vi "Start.vi"(0 "Address":string="localhost", 5 "Port":dbl=27015.0, 11 "error in (no error)":errorcluster) -> (4 "TecellaClient":refnum<class "TecellaClient.lvclass">, 6 "isAlive":bool, 8 "Is Simulated?":bool, 10 "Running?":bool, 15 "error out":errorcluster)   [LabVIEW 2009, in "TecellaClient.lvclass"]
uses:
  TecellaClient.lvclass
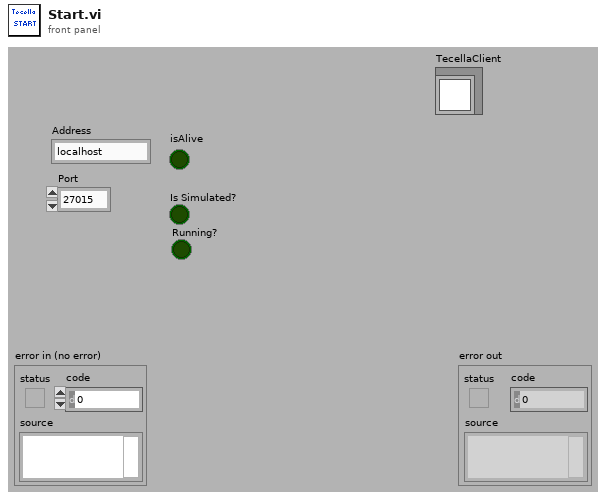
[diagram p1: front panel]
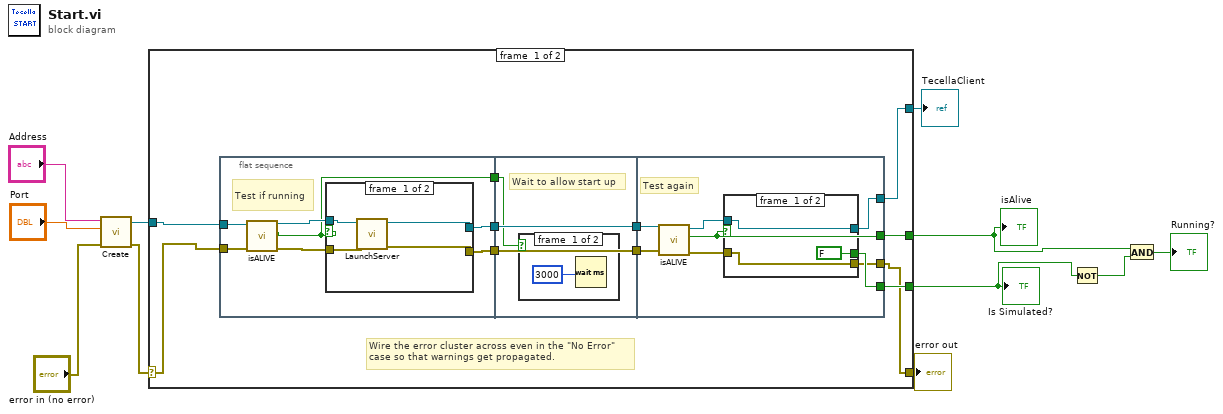
[diagram p0: block diagram]
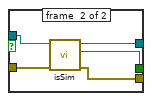
[diagram p4: hidden frame]
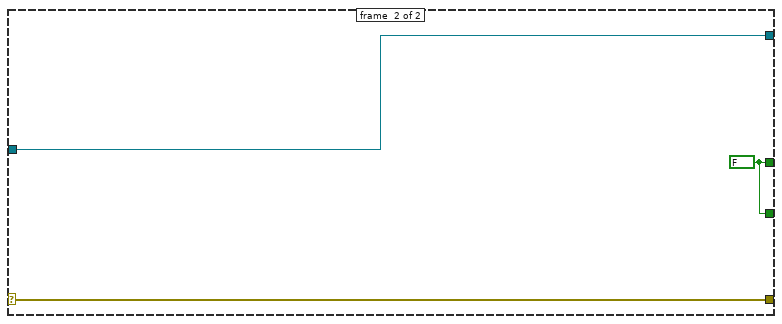
[diagram p5: hidden frame]
diagram:
  n1 = call "Create.vi"("error in (no error)"="error in (no error)", "Port"="Port", "Address"="Address") -> ("error out"=w8:errorcluster, "TecellaClient out"=w9:refnum<class "TecellaClient.lvclass">)  [unwired: 7 in]
  n2 = case shown="No Error" w8 {
    selector: w8 -> [w16 w57]
    tunnel: [w14 w57] -> w11
    tunnel: [w13 w58] -> w10
    tunnel: [w18 w56] -> w5
    tunnel: w9 -> [w17 w58]
    tunnel: [w15 w56] -> w4
    frame #0 {
      # "Wire the error cluster across even in the \"No Error\"\ncase so that warnings get propagated."
      n3 = flat-sequence {
        tunnel: [w29] -> w22
        tunnel: [w28] -> w21
        tunnel: w17 -> [w25]
        tunnel: w16 -> [w24]
        tunnel: [w23] -> w12
        tunnel: w22 -> [w38]
        tunnel: [w38] -> w20
        tunnel: w21 -> [w37]
        tunnel: [w37] -> w19
        tunnel: w12 -> [w36]
        tunnel: [w45] -> w18
        tunnel: w20 -> [w47]
        tunnel: w19 -> [w46]
        tunnel: [w44] -> w15
        tunnel: [w42] -> w14
        tunnel: [w41] -> w13
        frame #0 {
          # "Test if running"
          n4 = call-dynamic "isALIVE.vi"("error in (no error)"=w24, "TecellaClient in"=w25) -> ("error out"=w26:errorcluster, "Boolean"=w23:bool, "TecellaClient out"=w27:refnum<class "TecellaClient.lvclass">)  [unwired: 7 in]
          n5 = case shown="False" w23 {
            tunnel: [w32 w35] -> w29
            tunnel: [w33 w34] -> w28
            tunnel: w27 -> [w31 w35]
            tunnel: w26 -> [w30 w34]
            frame #0 {
              n6 = call-dynamic "LaunchServer.vi"("error in (no error)"=w30, "TecellaClient in"=w31) -> ("error out"=w33:errorcluster, "TecellaClient out"=w32:refnum<class "TecellaClient.lvclass">)  [unwired: 8 in]
            }
            frame #1 {
            }
          }
        }
        frame #1 {
          # "Wait to allow start up"
          n7 = case shown="False" w36 {
            frame #0 {
              n8 = Wait (ms)(milliseconds to wait=u32 3000) -> ()  [unwired: 1 out]
            }
            frame #1 {
            }
          }
        }
        frame #2 {
          # "Test again"
          n9 = call-dynamic "isALIVE.vi"("error in (no error)"=w46, "TecellaClient in"=w47) -> ("error out"=w43:errorcluster, "Boolean"=w45:bool, "TecellaClient out"=w40:refnum<class "TecellaClient.lvclass">)  [unwired: 7 in]
          n10 = case shown="False" w45 {
            tunnel: [FALSE ("Is Simulated?") w55] -> w44
            tunnel: w43 -> [w49 w54]
            tunnel: [w49 w53] -> w42
            tunnel: [w50 w52] -> w41
            tunnel: w40 -> [w50 w51]
            frame #0 {
            }
            frame #1 {
              n11 = call-dynamic "isSim.vi"("error in (no error)"=w54, "TecellaClient in"=w51) -> ("error out"=w53:errorcluster, "Is Simulated?"=w55:bool, "TecellaClient out"=w52:refnum<class "TecellaClient.lvclass">)  [unwired: 7 in]
            }
          }
        }
      }
    }
    frame #1 {
      w56 = FALSE ("Boolean")
    }
  }
  "error out" <- w11
  "isAlive" <- w5
  "TecellaClient" <- w10
  "Is Simulated?" <- w4
  n12 = Not(x=w4) -> (.not. x?=w6:bool)
  n13 = And(x=w5, y=w6) -> (x .and. y?=→"Running?":bool)
